vi "QuadraticOptimization.vi"(8 "Bias Amplitude":dbl, 9 "Neg Metric":dbl, 10 "Initial Metric":dbl, 11 "Pos Metric":dbl) -> (3 "Opt Variable (compared to 0)":dbl)   [LabVIEW 2018]
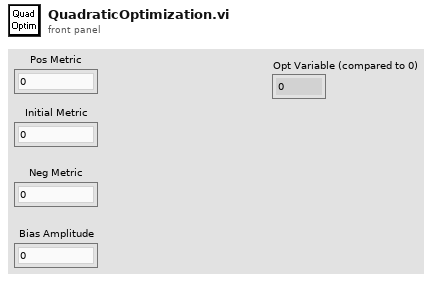
[diagram p1: front panel]
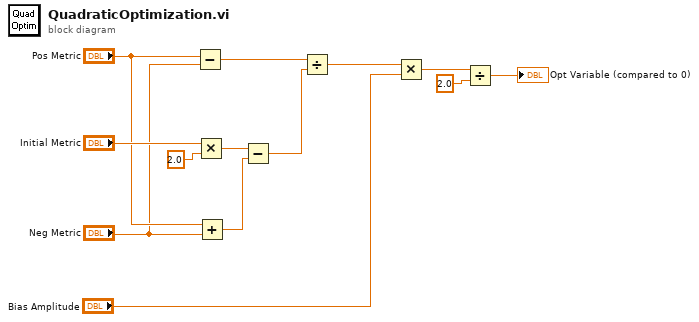
[diagram p0: block diagram]
diagram:
  n1 = Subtract(x="Pos Metric", y="Neg Metric") -> (x-y=w8:dbl)
  n2 = Multiply(x="Initial Metric", y=2.0) -> (x*y=w10:dbl)
  n3 = Add(x="Pos Metric", y="Neg Metric") -> (x+y=w9:dbl)
  n4 = Subtract(x=w10, y=w9) -> (x-y=w7:dbl)
  n5 = Divide(x=w8, y=w7) -> (x/y=w5:dbl)
  n6 = Multiply(x=w5, y="Bias Amplitude") -> (x*y=w3:dbl)
  n7 = Divide(x=w3, y=2.0) -> (x/y=→"Opt Variable (compared to 0)":dbl)
